vi "Configure.vi"(5 "Experimenter":string(combo)="Unselected", 7 "Subject":string(combo)="Testing", 8 "error in (no error)":errorcluster, 9 "Sample Lines":tag[](array[tag])=["/Dev3/ai/StartTrigger", "/Dev1/PXI_Trig4", "/4498_1/ai/StartTrigger", "/Dev1/PXI_Trig5", "/Dev1/PFI8"], 10 "DAQmx Device Name":tag="6608", 11 "TimeStamper in":refnum<class "TimeStamper.lvclass">) -> (0 "error out":errorcluster, 3 "TimeStamper out":refnum<class "TimeStamper.lvclass">)   [LabVIEW 2014, in "TimeStamper.lvclass"]
uses:
  TimeStamper.lvclass
  TimeStamper.lvclass/TimeStamper.ctl
  <vilib>/DAQmx/create/channels.llb/DAQmx Create Channel (CI-Count Edges).vi
  <vilib>/DAQmx/configure/timing.llb/DAQmx Timing (Sample Clock).vi
  <vilib>/Utility/config.llb/Read Key (I32).vi
  <resource>/objmgr/daqmx.rc
  <vilib>/Utility/config.llb/NI_LVConfig.lvlib
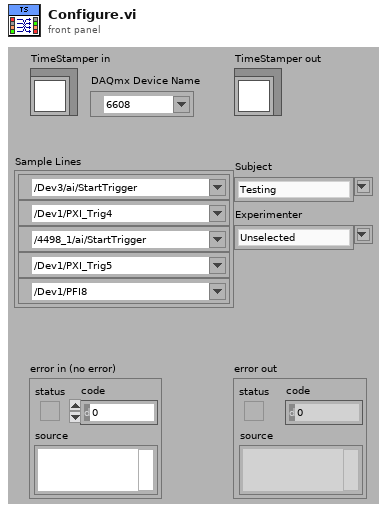
[diagram p1: front panel]
types:
  T1 = typedef "NI_LVConfig.lvlib/Config Data RefNum.ctl" = refnum<k1>
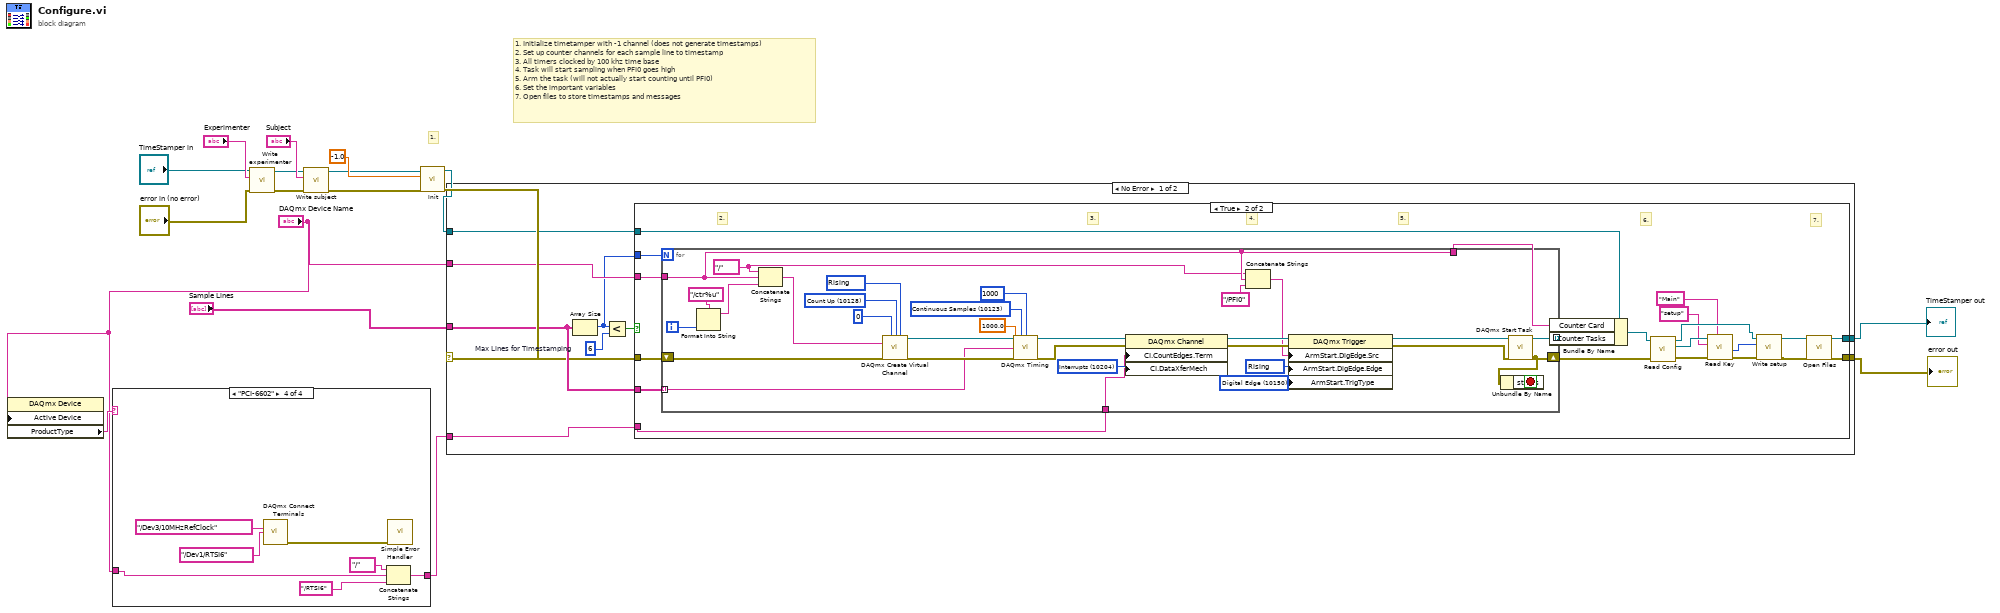
[diagram p0: block diagram]
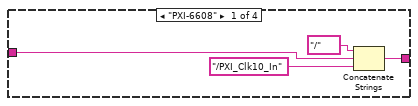
[diagram p2: hidden frame]
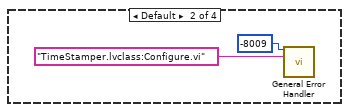
[diagram p3: hidden frame]
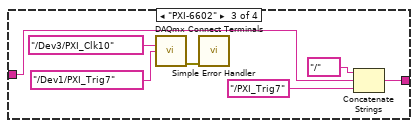
[diagram p4: hidden frame]
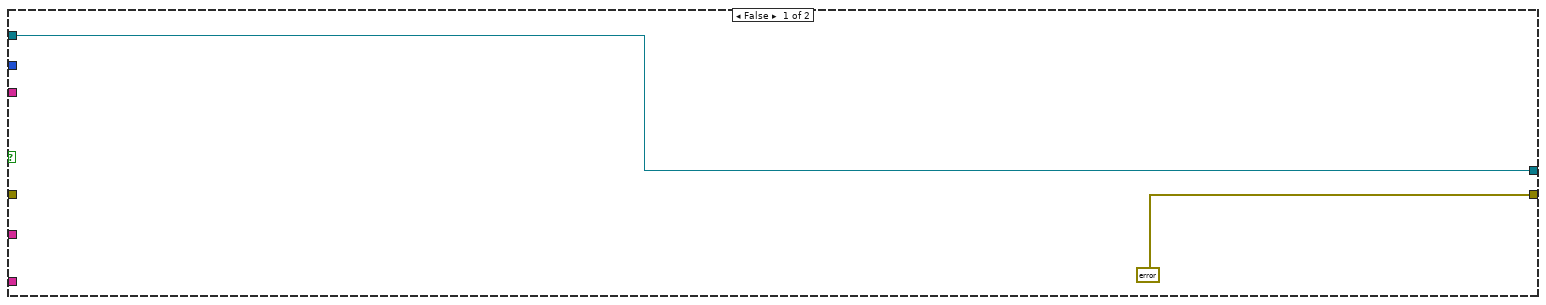
[diagram p5: hidden frame]
diagram:
  # "1. Initialize timetamper with -1 channel (does not generate timestamps)\n2. Set up counter channels for each sample line to timestamp\n3. All timers clocked by 100 khz time base\n4. Task will start sampling when PFI0 goes high\n5. Arm the task (will not actually start counting until PFI0)\n6. Set the important variables\n7. Open files to store timestamps and messages"
  # "1."
  n1 = property class="DAQmx Device"("Active Device"="DAQmx Device Name") -> ("ProductType"=w6:string)  [unwired: 2 in, 2 out]
  n2 = case shown="\"PCI-6602\"" w6 {
    tunnel: "DAQmx Device Name" -> [w19 _ w28 w33]
    tunnel: [w18 _ w25 w32] -> w4
    frame "PXI-6608" {
      n3 = Concatenate Strings(tag "/" ("string"), w19, "/PXI_Clk10_In" ("string")) -> (w18:string)
    }
    frame Default {
      n4 = call <vilib>:"General Error Handler.vi"("[error code] (0)"=-8009, "[error source] (\" \")"="TimeStamper.lvclass:Configure.vi" ("[error source] (\" \")")) -> ()  [unwired: 9 in, 5 out]
    }
    frame "PXI-6602" {
      n5 = call <vilib>:"DAQmx Connect Terminals.vi"("source terminal"=tag "/Dev3/PXI_Clk10", "destination terminal"=tag "/Dev1/PXI_Trig7") -> ("error out"=w24:errorcluster)  [unwired: 13 in]
      n6 = call <vilib>:"Simple Error Handler.vi"("error in (no error)"=w24) -> ()  [unwired: 4 in, 5 out]
      n7 = Concatenate Strings(tag "/" ("string"), w28, "/PXI_Trig7" ("string")) -> (w25:string)
    }
    frame "PCI-6602" {
      n8 = call <vilib>:"DAQmx Connect Terminals.vi"("source terminal"=tag "/Dev3/10MHzRefClock", "destination terminal"=tag "/Dev1/RTSI6") -> ("error out"=w31:errorcluster)  [unwired: 13 in]
      n9 = Concatenate Strings(tag "/" ("string"), w33, "/RTSI6" ("string")) -> (w32:string)
      n10 = call <vilib>:"Simple Error Handler.vi"("error in (no error)"=w31) -> ()  [unwired: 4 in, 5 out]
    }
  }
  n11 = call-dynamic "Write experimenter.vi"("error in (no error)"="error in (no error)", "experimenter"="Experimenter", "TimeStamper in"="TimeStamper in") -> ("error out"=w11:errorcluster, "TimeStamper out"=w12:refnum<class "TimeStamper.lvclass">)  [unwired: 7 in]
  n12 = call-dynamic "Write subject.vi"("error in (no error)"=w11, "subject"="Subject", "TimeStamper in"=w12) -> ("error out"=w10:errorcluster, "TimeStamper out"=w9:refnum<class "TimeStamper.lvclass">)  [unwired: 7 in]
  n13 = call-dynamic "Init.vi"("error in (no error)"=w10, "Channel"=-1.0, "AcquistionObject in"=w9) -> ("error out"=w17:errorcluster, "AcquistionObject out"=w15:refnum<class "TimeStamper.lvclass">)  [unwired: 7 in]
  n14 = case shown="No Error" w17 {
    selector: w17 -> [w42 w103]
    tunnel: [w41 w103] -> w3
    tunnel: [w39 w102] -> w2
    tunnel: w15 -> [w40 w102]
    tunnel: "Sample Lines" -> [w43 _]
    tunnel: "DAQmx Device Name" -> [w45 _]
    tunnel: w4 -> [w38 _]
    frame No Error {
      w47 = 6  # Max Lines for Timestamping
      n15 = Array Size(array=w43) -> (size(s)=w44:i32)
      n16 = Less?(x=w44, y=w47) -> (x < y?=w46:bool)
      n17 = case shown="True" w46 {
        tunnel: w45 -> [_ w65]
        tunnel: w44 -> [_ w70]
        tunnel: w43 -> [_ w69]
        tunnel: w42 -> [_ w68]
        tunnel: [errorcluster {"status"=TRUE, "code"=-150, "source"="Cannot initialize that many timestamped lines."} ("error IO") w63] -> w41
        tunnel: w40 -> [w49 w67]
        tunnel: [w49 w62] -> w39
        tunnel: w38 -> [_ w50]
        frame False {
        }
        frame True {
          # "6."
          # "7."
          # "5."
          # "4."
          # "3."
          # "2."
          n18 = for {
            N: w70 -> [_]
            tunnel: w65 -> [w77]
            tunnel: w69 -> [w82] mode=indexing
            shift-right: [w75] -> w54
            shift-left: w68 -> [w81]
            tunnel: [w80] -> w66 mode=indexing
            tunnel: [w77] -> w64
            tunnel: w50 -> [w71]
            i -> [w100]
            stop <- w74 stop-if-true
            w76 = tag "/" ("string")
            w84 = 10204 items=["DMA"=10054, "Interrupts"=10204, "Programmed I/O"=10264, "USB Bulk"=12590] ("CI.DataXferMech")
            w85 = 10150 items=["Digital Edge"=10150, "None"=10230] ("ArmStart.TrigType")
            w86 = 10280 items=["Rising"=10280, "Falling"=10171] ("ArmStart.DigEdge.Edge")
            w93 = 10123 items=["Finite Samples"=10178, "Continuous Samples"=10123, "Hardware Timed Single Point"=12522] ("sample mode")
            w96 = 10280 items=["Rising"=10280, "Falling"=10171] ("edge")
            w97 = 10128 items=["Count Up"=10128, "Count Down"=10124, "Externally Controlled"=10326] ("count direction")
            n19 = Format Into String(format string="/ctr%u", w100) -> (resulting string=w99:string)  [unwired: 2 in, 1 out]
            n20 = Concatenate Strings(w76, w77, w99) -> (w83:string)
            n21 = call-poly <vilib>:"DAQmx Create Virtual Channel.vi"("initial count"=0, "count direction"=w97, "edge"=w96, "counter"=w83, "error in"=w81) -> ("task out"=w95:refnum<k21>, "error out"=w94:errorcluster)  [unwired: 9 in]
            n22 = call-poly <vilib>:"DAQmx Timing.vi"("task/channels in"=w95, "sample mode"=w93, "samples per channel"=1000, "rate"=1000.0, "source"=w82, "error in"=w94) -> ("task out"=w89:refnum<k21>, "error out"=w90:errorcluster)  [unwired: 8 in]
            n23 = property class="DAQmx Channel"(reference=w89, error in=w90, "CI.CountEdges.Term"=w71, "CI.DataXferMech"=w84) -> (reference out=w88:refnum<k21>, error out=w87:errorcluster)
            n24 = Concatenate Strings(w76, w77, "/PFI0" ("string")) -> (w78:string)
            n25 = property class="DAQmx Trigger"(reference=w88, error in=w87, "ArmStart.DigEdge.Src"=w78, "ArmStart.DigEdge.Edge"=w86, "ArmStart.TrigType"=w85) -> (reference out=w73:refnum<k21>, error out=w72:errorcluster)
            n26 = call <vilib>:"DAQmx Start Task.vi"("task/channels in"=w73, "error in"=w72) -> ("task out"=w80:refnum<k21>, "error out"=w75:errorcluster)  [unwired: 12 in]
            n27 = Unbundle By Name(w75) -> ("status"=w74:bool)
          }
          n28 = Bundle By Name(cluster=w67, "Counter Card"=w64, "Counter Tasks"=w66) -> (w53:refnum<class "TimeStamper.lvclass">)
          n29 = call-dynamic "Read Config.vi"("error in (no error)"=w54, "AcquistionObject in"=w53) -> ("error out"=w58:errorcluster, "config data"=w57:T1, "AcquistionObject out"=w61:refnum<class "TimeStamper.lvclass">)  [unwired: 7 in]
          n30 = call-poly <vilib>:"Read Key.vi"("section"="Main", "error in (no error)"=w58, "key"="setup", "refnum"=w57) -> ("error out"=w59:errorcluster, "value"=w60:i32)  [unwired: 4 in, 2 out]
          n31 = call-dynamic "Write setup.vi"("error in (no error)"=w59, "setup"=w60, "TimeStamper in"=w61) -> ("error out"=w51:errorcluster, "TimeStamper out"=w52:refnum<class "TimeStamper.lvclass">)  [unwired: 7 in]
          n32 = call-dynamic "Open Files.vi"("error in (no error)"=w51, "TimeStamper in"=w52) -> ("error out"=w63:errorcluster, "TimeStamper out"=w62:refnum<class "TimeStamper.lvclass">)  [unwired: 8 in]
        }
      }
    }
    frame Error {
    }
  }
  "error out" <- w3
  "TimeStamper out" <- w2
